vi "S7COMM - Evaluate Setup Communication Response.vi"(8 "error in (no error)":errorcluster, 10 "S7 PDU":T1 format="0x%02x") -> (0 "error out":errorcluster)   [LabVIEW 2014, in "S7NetCom.lvclass"]
doc: "____\nCopyright (c) 2019 Hampel Software Engineering (HSE), released under BSD license. More info can be found on https://dokuwiki.hampel-soft.com/code/hse/s7netcom. Original code published by Marc Christenson, Sisu Devices."
uses:
  S7NetCom.lvclass
  Controls/S7NetCom_HexByteArray.ctl
  Controls/S7NetCom_HexByte.ctl
  S7COMM - Message Types--ring.ctl
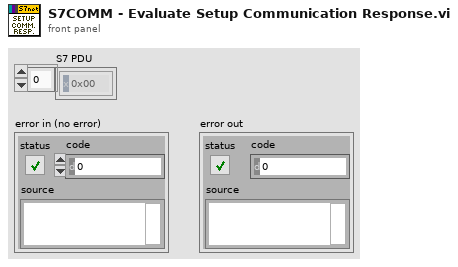
[diagram p1: front panel]
types:
  T1 = typedef "S7NetCom.lvclass/S7NetCom_HexByteArray.ctl" = T2[]
  T2 = typedef "S7NetCom.lvclass/S7NetCom_HexByte.ctl" = u8
  T3 = typedef "S7NetCom.lvclass/S7COMM - Message Types--ring.ctl" = u8
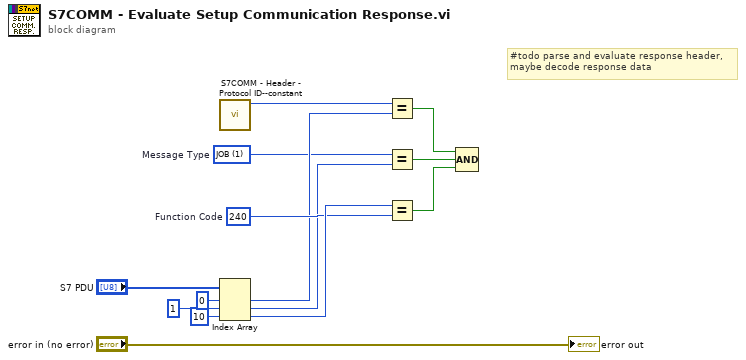
[diagram p0: block diagram]
diagram:
  w12 = T2 240  # Function Code
  w2 = T3 1 items=["JOB"=1, "ACK"=2, "ACK_DATA"=3, "USERDATA"=7]  # Message Type
  # "#todo parse and evaluate response header,\nmaybe decode response data"
  n1 = call "S7COMM - Header - Protocol ID--constant.vi"() -> ("Protocol ID"=w5:u8)  [unwired: 11 in]
  n2 = Index Array(array="S7 PDU", index #1=0 ("index"), index #2=1 ("index"), index #3=10 ("index")) -> (element #1=w4:T2, element #2=w3:T2, element #3=w13:T2)
  n3 = Equal?(x=w5, y=w4) -> (x = y?=w1:bool)
  n4 = Equal?(x=w2, y=w3) -> (x = y?=w11:bool)
  n5 = Equal?(x=w13, y=w12) -> (x = y?=w10:bool)
  n6 = Compound Arithmetic op=AND(w1, w11, w10) -> ()  [unwired: 1 out]
  "error out" <- "error in (no error)"
